vi "BRig_dataExp_T_ENL2_min.vi"() -> (2 "output_T_ENL2_min":i32)   [LabVIEW 2014]
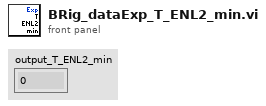
[diagram p1: front panel]
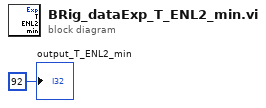
[diagram p0: block diagram]
diagram:
  "output_T_ENL2_min" <- 92 ("output_iBlock")
